vi "Process File.vi"(8 "error in (no error)":errorcluster, 10 "File":refnum<class "Acquired Result.lvclass">, 11 "Lockin Processor in":refnum<class "Lockin Processor.lvclass">) -> (0 "error out":errorcluster, 2 "File out":refnum<class "Acquired Result.lvclass">, 3 "Lockin Processor out":refnum<class "Lockin Processor.lvclass">)   [LabVIEW 2016, in "Lockin Processor.lvclass"]
uses:
  Lockin Processor.lvclass
  NHMFL_Core/Libraries/Instruments/Results/Acquired Result/Acquired Result.lvclass
  Lockin Processor.lvclass/Lockin Processor.ctl
  Read Lockin Processor Configuration.vi
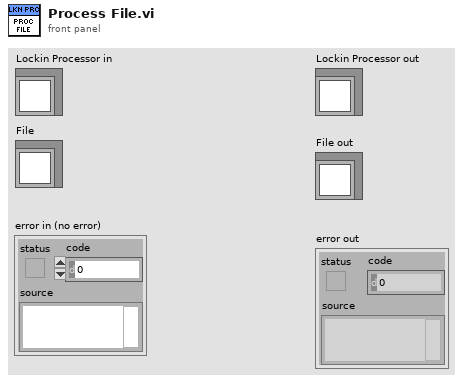
[diagram p1: front panel]
types:
  T1 = typedef "Lockin Processor Configuration.ctl" = cluster{"Time constant":dbl, "Signal channels":string[], "Group":string, "X channel":string, "Live update":bool, "Phases":dbl[], "Harmonics":i32[]}
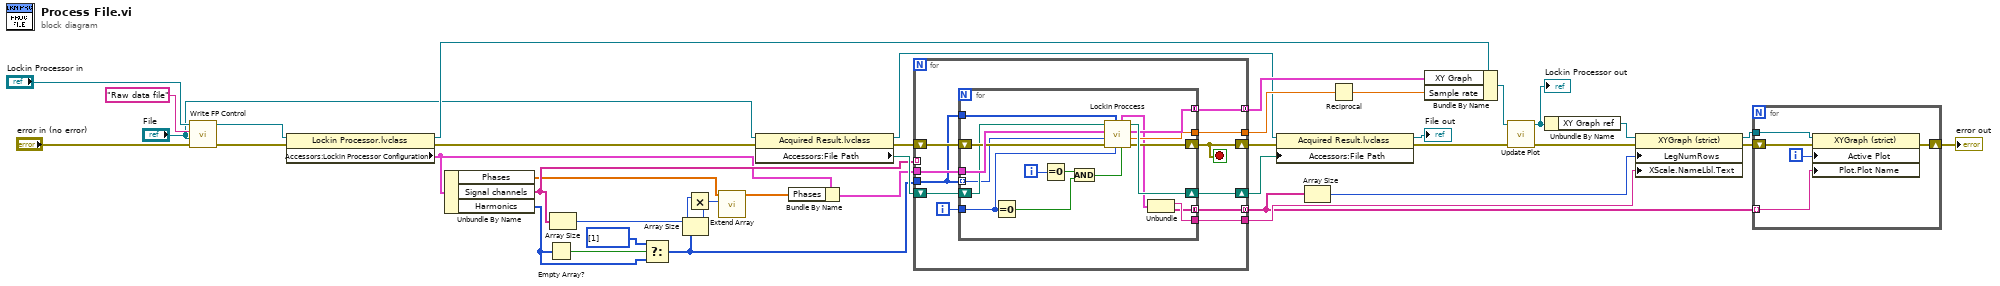
[diagram p0: block diagram]
diagram:
  n1 = call-dynamic "Write FP Control.vi"("error in (no error)"="error in (no error)", "Control Value"="File", "Control Name"="Raw data file", "Measure Object in"="Lockin Processor in") -> ("error out"=w36:errorcluster, "Measure Object out"=w38:refnum<class "Lockin Processor.lvclass">)  [unwired: 6 in]
  n2 = property class="Lockin Processor.lvclass"(reference=w38, error in=w36) -> (reference out=w35:refnum<class "Lockin Processor.lvclass">, error out=w14:errorcluster, "Accessors:Lockin Processor Configuration"=w11:T1)
  n3 = Unbundle By Name(w11) -> ("Phases"=w8:dbl[], "Signal channels"=w12:string[], "Harmonics"=w5:i32[])
  n4 = Empty Array?(array=w5) -> (empty?=w7:bool)
  n5 = Array Size(array=w12) -> (size(s)=w3:i32)
  n6 = Select(t=i32[] [1] ("Harmonics"), s=w7, f=w5) -> (s? t:f=w2:i32[])
  n7 = Array Size(array=w2) -> (size(s)=w1:i32)
  n8 = Multiply(x=w3, y=w1) -> (x*y=w4:i32)
  n9 = call "Extend Array.vi"("Extend to size"=w4, "Array in"=w8) -> ("Array out"=w9:dbl[])  [unwired: 8 in, 1 out]
  n10 = property class="Acquired Result.lvclass"(reference="File", error in=w14) -> (reference out=w21:refnum<class "Acquired Result.lvclass">, error out=w13:errorcluster, "Accessors:File Path"=w19:path)
  n11 = Bundle By Name(cluster=w11, "Phases"=w9) -> (w10:T1)
  n12 = for {
    shift-right: [w47] -> w18
    shift-left: w19 -> [w48]
    shift-right: [w44] -> w15
    shift-left: w13 -> [w49]
    tunnel: w10 -> [w51]
    tunnel: w12 -> [_] mode=indexing
    tunnel: [w46] -> w34 mode=concatenating
    tunnel: [w45] -> w32
    tunnel: [w42] -> w25 mode=concatenating
    tunnel: [w43] -> w27
    tunnel: w2 -> [w41]
    i -> [w50]
    stop <- w44 stop-if-true
    n13 = for {
      tunnel: w51 -> [w68]
      tunnel: w50 -> [w59]
      tunnel: [w64] -> w46 mode=concatenating
      tunnel: [w63] -> w45
      shift-right: [w62] -> w44
      shift-left: w49 -> [w67]
      shift-right: [w65] -> w47
      shift-left: w48 -> [w66]
      tunnel: w41 -> [w61] mode=indexing
      tunnel: [w54] -> w43
      tunnel: [w53] -> w42 mode=concatenating
      tunnel: w41 -> [w52]
      i -> [w60]
      n14 = Equal To 0?(x=w59) -> (x = 0?=w57:bool)
      n15 = Equal To 0?(x=w60) -> (x = 0?=w58:bool)
      n16 = And(x=w58, y=w57) -> (x .and. y?=w56:bool)
      n17 = call "Lockin Proccess.vi"("First call"=w56, "CH index"=w59, "Harmonics"=w52, "Error In"=w67, "Harmonic"=w61, "User configuration"=w68, "Signal file"=w66) -> ("Error Out"=w62:errorcluster, "dt"=w63:dbl, "XY Graph"=w64:cluster{dbl[], "Y":dbl[]}[], "Signal file out"=w65:path, "Signal names"=w55:cluster{"Signal Name":string, string[]})
      n18 = Unbundle(w55) -> ("Signal Name"=w54:string, w53:string[])
    }
  }
  n19 = property class="Acquired Result.lvclass"(reference=w21, error in=w15, "Accessors:File Path"=w18) -> (reference out=→"File out":refnum<class "Acquired Result.lvclass">, error out=w16:errorcluster)
  n20 = Array Size(array=w25) -> (size(s)=w28:i32)
  n21 = Reciprocal(x=w32) -> (1/x=w31:dbl)
  n22 = Bundle By Name(cluster=w35, "XY Graph"=w34, "Sample rate"=w31) -> (w33:refnum<class "Lockin Processor.lvclass">)
  n23 = call-dynamic "Update Plot.vi"("error in (no error)"=w16, "Lockin Processor in"=w33) -> ("error out"=w26:errorcluster, "Lockin Processor out"=w30:refnum<class "Lockin Processor.lvclass">)  [unwired: 8 in]
  "Lockin Processor out" <- w30
  n24 = Unbundle By Name(w30) -> ("XY Graph ref"=w29:refnum<vi>)
  n25 = property class="XYGraph (strict)"(reference=w29, error in=w26, "LegNumRows"=w28, "XScale.NameLbl.Text"=w27) -> (reference out=w22:refnum<vi>, error out=w24:errorcluster)
  n26 = for {
    tunnel: w25 -> [w73] mode=indexing
    shift-right: [w70] -> w23
    shift-left: w24 -> [w71]
    tunnel: w22 -> [w69]
    i -> [w72]
    n27 = property class="XYGraph (strict)"(reference=w69, error in=w71, "Active Plot"=w72, "Plot.Plot Name"=w73) -> (error out=w70:errorcluster)  [unwired: 1 out]
  }
  "error out" <- w23
